vi "Set Properties (String Array).vi"(8 "error in (no error)":errorcluster, 9 "values (string)":string[](array[string]), 10 "names":string[](array[string]), 11 "CycloneDX JSON in":refnum<class "CycloneDX JSON.lvclass">) -> (0 "error out":errorcluster, 3 "CycloneDX JSON out":refnum<class "CycloneDX JSON.lvclass">)   [LabVIEW 2017, in "LabVIEW CycloneDX SBOM.lvlib" / "CycloneDX JSON.lvclass"]
doc: "Adds property items (name-value pairs) at the specified JSON path."
uses:
  CycloneDX JSON.lvclass
  Name Value Pair.ctl
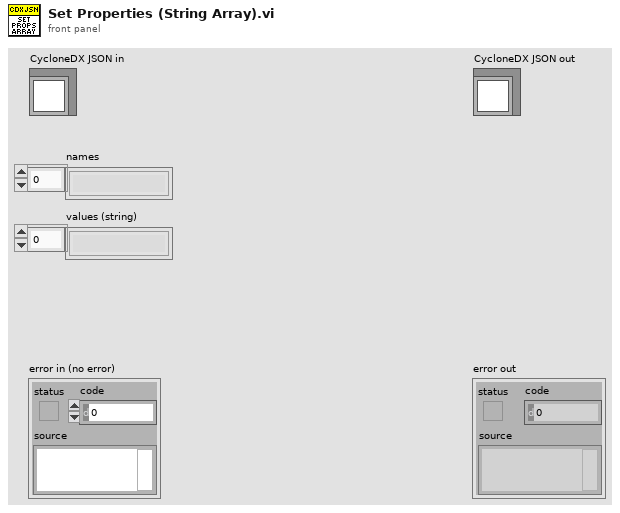
[diagram p1: front panel]
types:
  T1 = typedef "LabVIEW CycloneDX SBOM.lvlib/CycloneDX JSON.lvclass/Name Value Pair.ctl" = cluster{"name":string, "value":string}
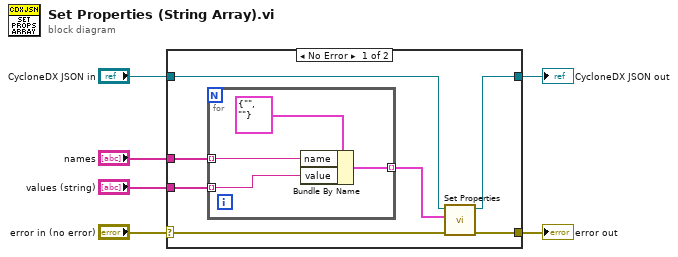
[diagram p0: block diagram]
diagram:
  n1 = case shown="No Error" "error in (no error)" {
    selector: "error in (no error)" -> [w12 w19]
    tunnel: [w11 w19] -> w5
    tunnel: [w10 w18] -> w3
    tunnel: "CycloneDX JSON in" -> [w13 w18]
    tunnel: "names" -> [w9 _]
    tunnel: "values (string)" -> [w8 _]
    frame No Error {
      n2 = for {
        tunnel: w9 -> [w15] mode=indexing
        tunnel: w8 -> [w14] mode=indexing
        tunnel: [w16] -> w7 mode=indexing
        n3 = Bundle By Name(cluster=T1 {"name"="", "value"=""} ("Name Value Pair"), "name"=w15, "value"=w14) -> (w16:T1)
      }
      n4 = call-dynamic "Set Properties.vi"("error in (no error)"=w12, "Properties"=w7, "CycloneDX JSON in"=w13) -> ("error out"=w11:errorcluster, "CycloneDX JSON out"=w10:refnum<class "CycloneDX JSON.lvclass">)  [unwired: 7 in]
    }
    frame Error {
    }
  }
  "error out" <- w5
  "CycloneDX JSON out" <- w3
